vi "RigidFieldOffset.vi"(1 "Downward's Hc":dbl, 2 "Upward's Hc":dbl) -> (0 "Rigid Field offset":dbl)   [LabVIEW 2019]
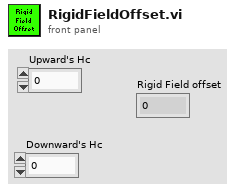
[diagram p1: front panel]
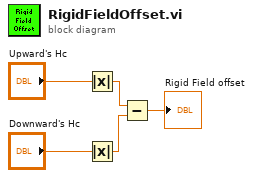
[diagram p0: block diagram]
diagram:
  n1 = Absolute Value(x="Upward's Hc") -> (abs(x)=w5:dbl)
  n2 = Absolute Value(x="Downward's Hc") -> (abs(x)=w2:dbl)
  n3 = Subtract(x=w5, y=w2) -> (x-y=→"Rigid Field offset":dbl)
